vi "waveform array size.vi"(10 "Waveform":waveform(dbl)[](array[waveform])) -> (0 "min value":i32, 1 "max value":i32, 2 "Array":i32[](array[numeric]))   [LabVIEW 2020]
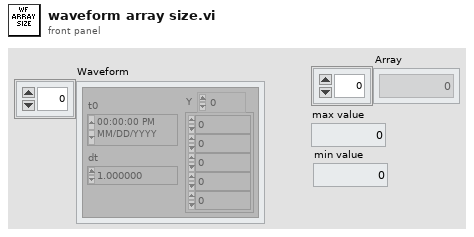
[diagram p1: front panel]
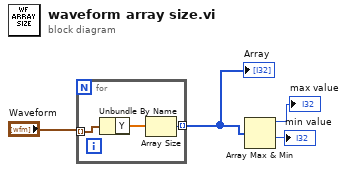
[diagram p0: block diagram]
diagram:
  n1 = for {
    tunnel: "Waveform" -> [w7] mode=indexing
    tunnel: [w5] -> w3 mode=indexing
    n2 = Unbundle By Name(w7) -> ("Y"=w6:dbl[])
    n3 = Array Size(array=w6) -> (size(s)=w5:i32)
  }
  "Array" <- w3
  n4 = Array Max & Min(array=w3) -> (max value=→"max value":i32, min value=→"min value":i32)  [unwired: 2 out]
